vi "7.2.vi"() -> ()   [LabVIEW 2017]
panel:
  out "min index(es)":i32
  out "x*y":dbl format="%#_21f"
  out "array":i32[](array[numeric])
  in  "String":string
  # "127900529"
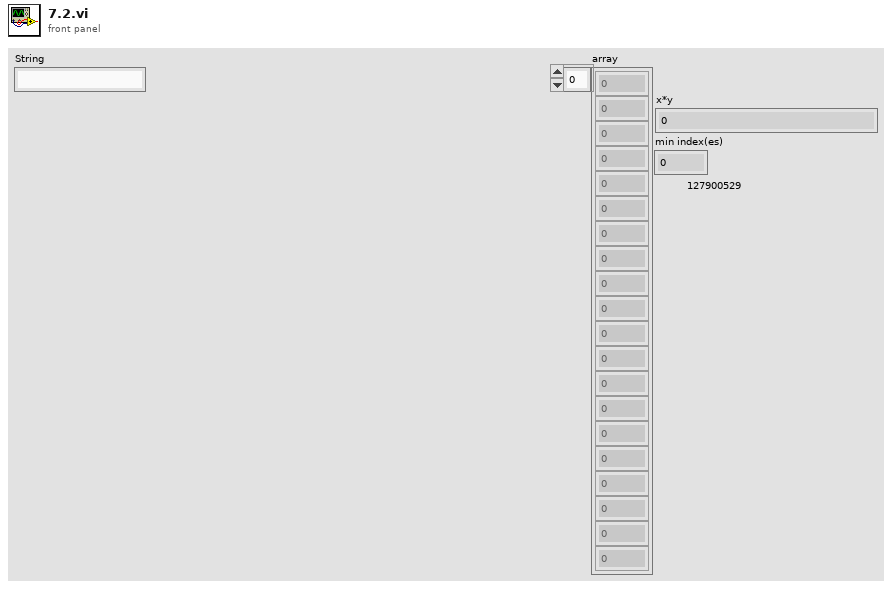
[diagram p1: front panel]
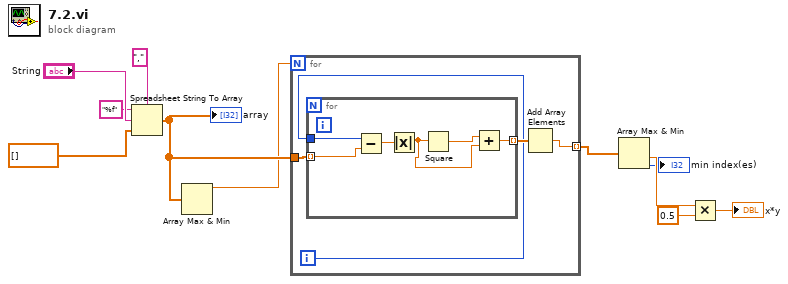
[diagram p0: block diagram]
diagram:
  n1 = Spreadsheet String To Array(delimiter (Tab)=",", format string="%f", spreadsheet string="String", array type (2D Dbl)=dbl[] []) -> (array=w7:dbl[])
  "array" <- w7
  n2 = Array Max & Min(array=w7) -> (max value=w6:dbl)  [unwired: 3 out]
  n3 = for {
    N: w6 -> [_]
    tunnel: w7 -> [w15]
    tunnel: [w14] -> w5 mode=indexing
    i -> [w12]
    n4 = for {
      tunnel: w15 -> [w21] mode=indexing
      tunnel: [w17] -> w13 mode=indexing
      tunnel: w12 -> [w16]
      n5 = Subtract(x=w16, y=w21) -> (x-y=w20:dbl)
      n6 = Absolute Value(x=w20) -> (abs(x)=w18:dbl)
      n7 = Square(x=w18) -> (x^2=w19:dbl)
      n8 = Add(x=w19, y=w18) -> (x+y=w17:dbl)
    }
    n9 = Add Array Elements(numeric array=w13) -> (sum=w14:dbl)
  }
  n10 = Array Max & Min(array=w5) -> (min value=w4:dbl, min index (indices)=→"min index(es)":i32)  [unwired: 2 out]
  n11 = Multiply(x=w4, y=0.5) -> (x*y=→"x*y":dbl)
